vi "ProcessIntegration.vi"(8 "error in (no error)":errorcluster, 9 "parent waveform":waveform(sgl), 10 "parent found":bool, 11 "virtual channel":T1) -> (0 "error out":errorcluster, 2 "integrated waveform":waveform(sgl), 3 "virtual channel out":T1)   [LabVIEW 2017, in "CmsVirtualChannel.lvlib"]
uses:
  <vilib>/addons/InsightCM/Devices/Shared/Cms/CmsVirtualChannel/CmsVirtualChannel.lvlib
  <vilib>/addons/InsightCM/Devices/Shared/Cms/CmsVirtualChannel/controls/VirtualChannel.ctl
  <vilib>/addons/InsightCM/Devices/Shared/Cms/CmsVirtualChannel/controls/Integration.ctl
  <vilib>/addons/InsightCM/Utilities/Analysis/Shared/controls/ConversionOp.ctl
  <vilib>/addons/InsightCM/Utilities/Analysis/Vibration/controls/LowPassFilterState.ctl
  <vilib>/addons/InsightCM/Utilities/Analysis/Vibration/controls/HighPassFilterState.ctl
  <vilib>/addons/InsightCM/Utilities/Analysis/Shared/AnalysisHelper.lvlib
  <vilib>/addons/InsightCM/Utilities/ChannelStatus/ChannelStatus.lvlib
  <vilib>/addons/InsightCM/Utilities/Analysis/Vibration/VibrationAnalysisFunctions.lvlib
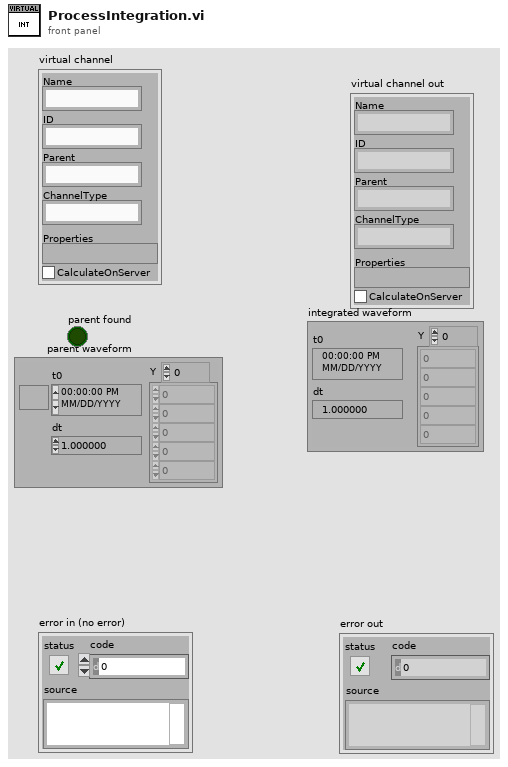
[diagram p1: front panel]
types:
  T1 = typedef "CmsVirtualChannel.lvlib/VirtualChannel.ctl" = cluster{"Name":string, "ID":string, "Parent":string, "ChannelType":string, "Properties":variant, "CalculateOnServer":bool}
  T2 = typedef "CmsVirtualChannel.lvlib/Integration.ctl" = cluster{"Conversion Op":T3, "Unit":string, "Parent Unit":string, "Single Integration Cutoff":dbl, "Double Integration Cutoff":dbl, "Lowpass Filter State":T4, "Highpass Filter State":T5, "Wfm Scale":sgl}
  T3 = typedef "AnalysisHelper.lvlib/ConversionOp.ctl" = enum16{"none", "singleInt", "doubleInt", "singleDiff", "doubleDiff"}
  T4 = typedef "VibrationAnalysisFunctions.lvlib/LowPassFilterState.ctl" = cluster{"designed":bool, "integration filter coefficients":cluster{"beta":dbl, "gamma":dbl, "alpha":dbl}, "state":cluster{"x(n-1) state":dbl, "y(n-1) state":dbl, "x(n-2) state":dbl, "y(n-2) state":dbl}}
  T5 = typedef "VibrationAnalysisFunctions.lvlib/HighPassFilterState.ctl" = cluster{"designed":bool, "IIR Filter Cluster":cluster{"filter structure":enum32{"IIR 2nd Order", "IIR 4th Order"}, "Reverse Coefficients":dbl[], "Forward Coefficients":dbl[]}, "Filter State":dbl[]}
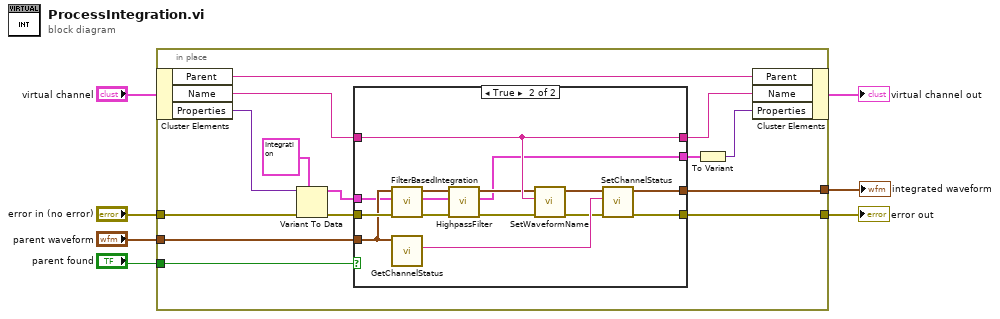
[diagram p0: block diagram]
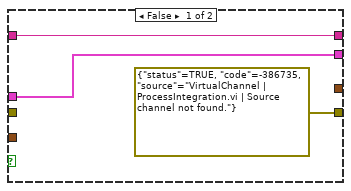
[diagram p2: hidden frame]
diagram:
  n1 = in-place {
    in-place-border: "error in (no error)" -> [w21]
    in-place-border: [w17] -> w4
    in-place-border: [w10] -> w3
    in-place-border: "parent waveform" -> [w9]
    in-place-border: "parent found" -> [w8]
    n2 = in-place-cluster #1("virtual channel") -> ("Parent"=w18:string, "Name"=w14:string, "Properties"=w12:variant)
    n3 = Variant To Data(error in=w21, type=T2 {"Conversion Op"=enum."singleInt", "Unit"="", "Parent Unit"="", "Single Integration Cutoff"=0.0, "Double Integration Cutoff"=0.0, "Lowpass Filter State"={"designed"=FALSE, "integration filter coefficients"={"beta"=0.0, "gamma"=0.0, "alpha"=0.0}, "state"={"x(n-1) state"=0.0, "y(n-1) state"=0.0, "x(n-2) state"=0.0, "y(n-2) state"=0.0}}, "Highpass Filter State"={"designed"=FALSE, "IIR Filter Cluster"={"filter structure"=enum."IIR 2nd Order", "Reverse Coefficients"=[], "Forward Coefficients"=[]}, "Filter State"=[]}, "Wfm Scale"=0.0} ("Integration"), Variant=w12) -> (data=w16:T2, error out=w19:errorcluster)
    n4 = case shown="True" w8 {
      tunnel: w19 -> [_ w38]
      tunnel: [errorcluster {"status"=TRUE, "code"=-386735, "source"="VirtualChannel | ProcessIntegration.vi | Source channel not found."} ("error in (no error)") w34] -> w17
      tunnel: w16 -> [w24 w27]
      tunnel: w9 -> [_ w29]
      tunnel: [w24 w25] -> w15
      tunnel: w14 -> [w23 w31]
      tunnel: [w23 w31] -> w13
      tunnel: [_ w35] -> w10
      frame False {
      }
      frame True {
        n5 = call <vilib>:"FilterBasedIntegration.vi"("error in (no error)"=w38, "Integration Properties in"=w27, "Waveform"=w29) -> ("error out"=w39:errorcluster, "Integration Properties out"=w26:T2, "Integrated Waveform"=w37:waveform(sgl))  [unwired: 6 in]
        n6 = call <vilib>:"GetChannelStatus.vi"("waveform in"=w29) -> ("channel status"=w33:string)  [unwired: 7 in, 3 out]
        n7 = call <vilib>:"HighpassFilter.vi"("error in (no error)"=w39, "Integration Properties in"=w26, "Waveform"=w37) -> ("error out"=w36:errorcluster, "Integration Properties out"=w25:T2, "Highpass Filtered Waveform"=w28:waveform(sgl))  [unwired: 6 in]
        n8 = call <vilib>:"SetWaveformName.vi"("error in (no error)"=w36, "Name"=w31, "Waveform in"=w28) -> ("error out"=w32:errorcluster, "Waveform out"=w30:waveform(sgl))  [unwired: 7 in]
        n9 = call <vilib>:"SetChannelStatus.vi"("error in (no error)"=w32, "Channel Status"=w33, "Waveform in"=w30) -> ("error out"=w34:errorcluster, "Waveform out"=w35:waveform(sgl))  [unwired: 7 in]
      }
    }
    n10 = To Variant(anything=w15) -> (Variant=w11:variant)
    n11 = in-place-cluster #1("Parent"=w18, "Name"=w13, "Properties"=w11) -> (→"virtual channel out":T1)
  }
  "error out" <- w4
  "integrated waveform" <- w3
